vi "createDocumentObjectByFileExtension.vi"(8 "error in (no error)":errorcluster, 10 "File Path":path) -> (0 "error out":errorcluster, 2 "File Path dup":path, 3 "Document out":refnum<class "Document.lvclass">)   [LabVIEW 2017, in "LabVIEW NPOI.lvlib" / "Document.lvclass"]
uses:
  Document.lvclass
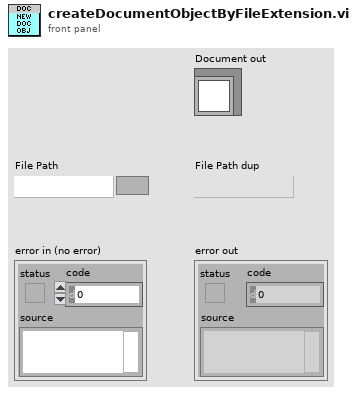
[diagram p1: front panel]
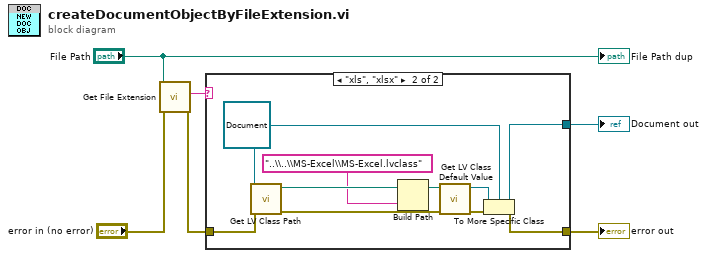
[diagram p0: block diagram]
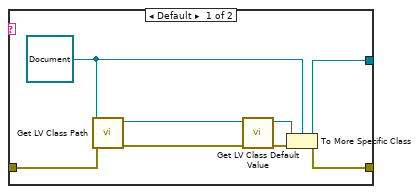
[diagram p2: hidden frame]
diagram:
  n1 = call <vilib>:"Get File Extension.vi"("error in (no error)"="error in (no error)", "file"="File Path") -> ("error out"=w2:errorcluster, "lowercase file extension"=w1:string)  [unwired: 5 in, 3 out]
  n2 = case shown="\"xls\", \"xlsx\"" w1 {
    tunnel: [w14 w24] -> w5
    tunnel: w2 -> [w13 w23]
    tunnel: [w12 w22] -> w6
    frame Default {
      w11 = refnum<class "Document.lvclass"> refnum ("LabVIEW NPOI.lvlib:Document.lvclass")
      n3 = call <vilib>:"Get LV Class Path.vi"("error in (no error)"=w13, "object"=w11) -> ("error out"=w10:errorcluster, "class path"=w9:path)  [unwired: 8 in]
      n4 = call <vilib>:"Get LV Class Default Value.vi"("error in (no error)"=w10, "class path"=w9) -> ("error out"=w8:errorcluster, "object"=w7:refnum<class>)  [unwired: 8 in]
      n5 = To More Specific Class(target class=w11, reference=w7, error in=w8) -> (specific class reference=w14:refnum<class "Document.lvclass">, error out=w12:errorcluster)
    }
    frame "xls", "xlsx" {
      w18 = refnum<class "Document.lvclass"> refnum ("LabVIEW NPOI.lvlib:Document.lvclass")
      n6 = call <vilib>:"Get LV Class Path.vi"("error in (no error)"=w23, "object"=w18) -> ("error out"=w21:errorcluster, "class path"=w17:path)  [unwired: 8 in]
      n7 = Build Path(base path=w17, name or relative path="..\\..\\MS-Excel\\MS-Excel.lvclass") -> (appended path=w16:path)
      n8 = call <vilib>:"Get LV Class Default Value.vi"("error in (no error)"=w21, "class path"=w16) -> ("error out"=w20:errorcluster, "object"=w19:refnum<class>)  [unwired: 8 in]
      n9 = To More Specific Class(target class=w18, reference=w19, error in=w20) -> (specific class reference=w24:refnum<class "Document.lvclass">, error out=w22:errorcluster)
    }
  }
  "error out" <- w6
  "Document out" <- w5
  "File Path dup" <- "File Path"
